vi "_L_SearchArray.vi"(2 "String":string) -> (0 "name or relative path":string)   [LabVIEW 2017]
panel:
  in  "Search Array":string[](array[string])=["Description", "Free text 1", "Free text 2", "Free text 3", "Name", "Unit", "Data type", "Free integer 1", "Free integer 2", "Free integer 3", "Free integer 4", "Free integer 5", "Free integer 6", "Free number 1", "Free number 2", "Free number 3", "Free number 4", "Free number 5", "Free number 6", "Maximum", "Minimum", "Author", "Title"]
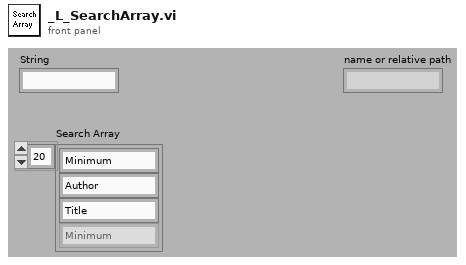
[diagram p1: front panel]
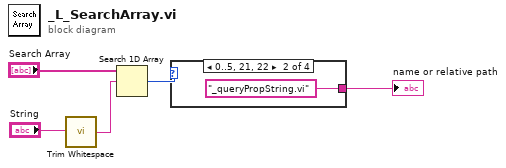
[diagram p0: block diagram]
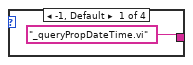
[diagram p2: hidden frame]
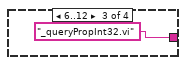
[diagram p3: hidden frame]
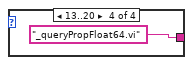
[diagram p4: hidden frame]
diagram:
  n1 = call <vilib>:"Trim Whitespace.vi"("string"="String") -> ("trimmed string"=w1:string)  [unwired: 1 in]
  n2 = Search 1D Array(1D array="Search Array", element=w1) -> (index of element=w4:i32)  [unwired: 1 in]
  n3 = case shown="0..5, 21, 22" w4 {
    tunnel: ["_queryPropDateTime.vi" ("name or relative path") "_queryPropString.vi" ("name or relative path") "_queryPropInt32.vi" ("name or relative path") "_queryPropFloat64.vi" ("name or relative path")] -> w5
    frame -1, Default {
    }
    frame 0..5, 21, 22 {
    }
    frame 6..12 {
    }
    frame 13..20 {
    }
  }
  "name or relative path" <- w5
